vi "Zaber A Series XY List.vi"() -> ()   [LabVIEW 2012]
doc: "This example moves a two-axis system through a list of co-ordinates. It uses the Move command as well as the Poll Until Idle library VI to cor-ordinate the timing of the movements with the two stages."
uses:
  <instrlib>/Zaber A Series/Zaber A Series.lvlib
panel:
  in  "Units (0: microsteps)":u16(ring) items=["microsteps", "microns", "millimeters", "inches"]
  in  "Movement Type (0: relative)":u16(ring) items=["relative", "absolute"]
  in  "Y-Axis Microstep Size (0)":dbl
  in  "XY Positions":string[][](table)
  in  "Y-Axis (02)":string="02"
  in  "X-Axis (01)":string="01"
  in  "X-Axis Microstep Size (0)":dbl
  in  "VISA resource name":refnum<visa-resource-name>
  # "(c) 2014 Zaber Technologies.  ALL RIGHTS RESERVED."
  # "This example demonstrates how you can move between co-ordinates. Before running, enter all of the XY points you'd like your stages to move to and the VISA resource name of your conenction. Make sure the units of your positions match the units dropdown. Also ensure that the Axis numbers correspond to your device numbers. Finally enter the microstep sizes of the devices if you are using something other than microsteps. This example could be easily expanded for XYZ positions."
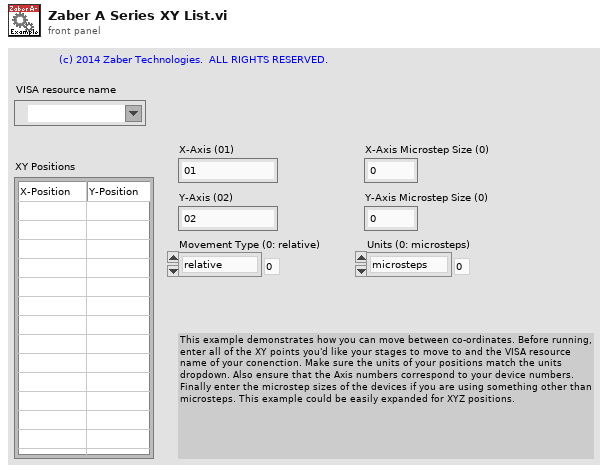
[diagram p1: front panel]
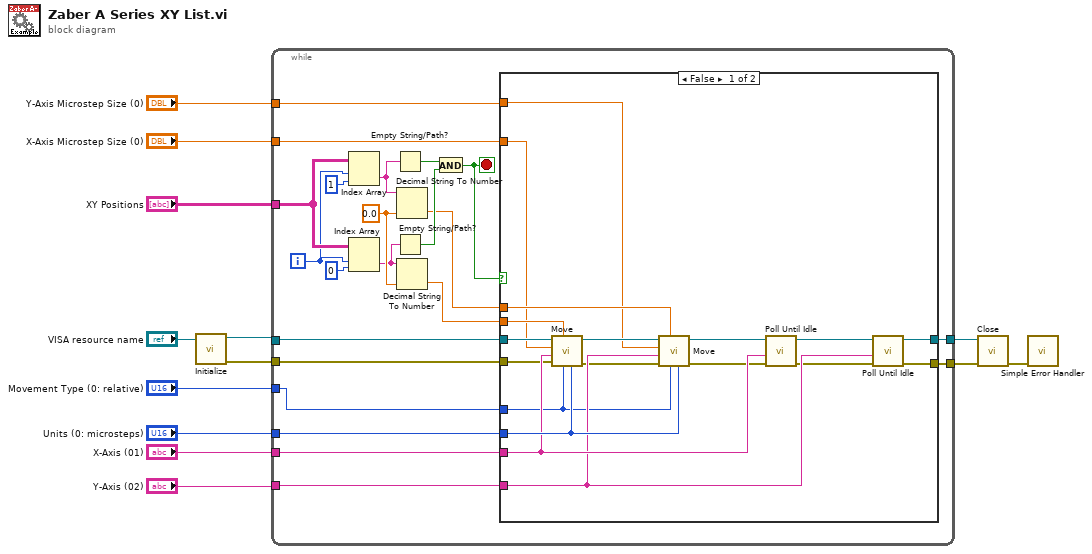
[diagram p0: block diagram]
diagram:
  n1 = call <instrlib>:"Initialize.vi"("VISA resource name"="VISA resource name") -> ("error out"=w6:errorcluster, "VISA resource name out"=w11:refnum<visa-resource-name>)  [unwired: 9 in]
  n2 = while {
    tunnel: w11 -> [w35]
    tunnel: "XY Positions" -> [w27]
    tunnel: "Units (0: microsteps)" -> [w22]
    tunnel: "Movement Type (0: relative)" -> [w21]
    tunnel: "Y-Axis (02)" -> [w20]
    tunnel: "X-Axis (01)" -> [w19]
    tunnel: w6 -> [w18]
    tunnel: [w17] -> w5
    tunnel: [w16] -> w4
    tunnel: "Y-Axis Microstep Size (0)" -> [w15]
    tunnel: "X-Axis Microstep Size (0)" -> [w14]
    i -> [w26]
    stop <- w24 stop-if-true
    w33 = 0.0
    n3 = Index Array(array=w27, index (row)=w26, index (col)=1 ("disabled index (col)")) -> (element=w34:string)
    n4 = Index Array(array=w27, index (row)=w26, index (col)=0 ("disabled index (col)")) -> (element=w32:string)
    n5 = Empty String/Path?(string/path=w34) -> (empty?=w29:bool)
    n6 = Empty String/Path?(string/path=w32) -> (empty?=w28:bool)
    n7 = Decimal String To Number(string=w34, default (0L)=w33) -> (number=w23:dbl)  [unwired: 1 in, 1 out]
    n8 = Decimal String To Number(string=w32, default (0L)=w33) -> (number=w25:dbl)  [unwired: 1 in, 1 out]
    n9 = And(x=w29, y=w28) -> (x .and. y?=w24:bool)
    n10 = case shown="False" w24 {
      tunnel: w22 -> [w53 _]
      tunnel: w35 -> [w44 w54]
      tunnel: w19 -> [w49 _]
      tunnel: w20 -> [w48 _]
      tunnel: w21 -> [w47 _]
      tunnel: w25 -> [w46 _]
      tunnel: w23 -> [w45 _]
      tunnel: w18 -> [w43 w55]
      tunnel: [w39 w55] -> w16
      tunnel: [w38 w54] -> w17
      tunnel: w15 -> [w37 _]
      tunnel: w14 -> [w36 _]
      frame False {
        n11 = call <instrlib>:"Move.vi"("Units (0: microsteps)"=w53, "Movement Type (0: relative)"=w47, "Move Distance (0)"=w46, "error in (no error)"=w43, "Device and Axis"=w49, "Microstep Size (0)"=w36, "VISA resource name"=w44) -> ("error out"=w42:errorcluster, "VISA resource name out"=w52:refnum<visa-resource-name>)  [unwired: 3 in]
        n12 = call <instrlib>:"Move.vi"("Units (0: microsteps)"=w53, "Movement Type (0: relative)"=w47, "Move Distance (0)"=w45, "error in (no error)"=w42, "Device and Axis"=w48, "Microstep Size (0)"=w37, "VISA resource name"=w52) -> ("error out"=w41:errorcluster, "VISA resource name out"=w51:refnum<visa-resource-name>)  [unwired: 3 in]
        n13 = call <instrlib>:"Poll Until Idle.vi"("error in (no error)"=w41, "Device and Axis"=w49, "VISA resource name"=w51) -> ("error out"=w40:errorcluster, "VISA resource name out"=w50:refnum<visa-resource-name>)  [unwired: 7 in]
        n14 = call <instrlib>:"Poll Until Idle.vi"("error in (no error)"=w40, "Device and Axis"=w48, "VISA resource name"=w50) -> ("error out"=w39:errorcluster, "VISA resource name out"=w38:refnum<visa-resource-name>)  [unwired: 7 in]
      }
      frame True {
      }
    }
  }
  n15 = call <instrlib>:"Close.vi"("error in (no error)"=w4, "VISA resource name"=w5) -> ("error out"=w3:errorcluster)  [unwired: 9 in]
  n16 = call <vilib>:"Simple Error Handler.vi"("error in (no error)"=w3) -> ()  [unwired: 4 in, 5 out]
